vi "BIN_PAQ_content2chunkDefs.vi"(8 "error in (no error)":errorcluster, 11 "Content":string) -> (0 "error out":errorcluster, 3 "Data segments":cluster{"Offset":u32, "Size":u32}[](array[cluster]))   [LabVIEW 2020, in "DBAL-BIN.lvclass"]
doc: "Get PAQ BIN file content and deliver into data chunk segment definitions"
uses:
  DBAL-BIN.lvclass
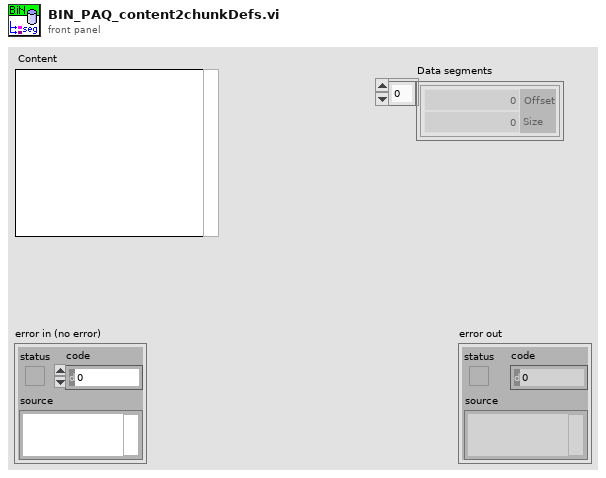
[diagram p1: front panel]
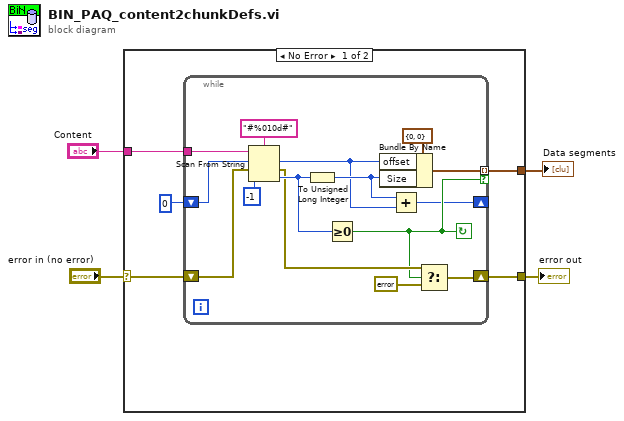
[diagram p0: block diagram]
diagram:
  n1 = case shown="No Error" "error in (no error)" {
    selector: "error in (no error)" -> [w7 w25]
    tunnel: [w6 w25] -> w3
    tunnel: "Content" -> [w9 _]
    tunnel: [w5 _] -> w1
    frame No Error {
      n2 = while {
        tunnel: w9 -> [w18]
        shift-right: [w12] -> _
        shift-left: u32 0 ("offset past scan") -> [w17]
        tunnel: [w22] -> w5 mode=indexing if=w13
        shift-right: [w15] -> w6
        shift-left: w7 -> [w21]
        stop <- w13 continue-if-true
        n3 = Scan From String(format string="#%010d#", input string=w18, initial scan location=w17, error in=w21, default 1=-1 ("default value 1")) -> (offset past scan=w10:u32, error out=w16:errorcluster, output 1=w19:i32)  [unwired: 1 out]
        n4 = To Unsigned Long Integer(number=w19) -> (unsigned 32bit integer=w11:u32)
        n5 = Greater Or Equal To 0?(x=w19) -> (x >= 0?=w13:bool)
        n6 = Bundle By Name(cluster=cluster{"offset":u32, "Size":u32} {"offset"=0, "Size"=0} ("Cluster"), "offset"=w10, "Size"=w11) -> (w22:cluster{"offset":u32, "Size":u32})
        n7 = Add(x=w11, y=w10) -> (x+y=w12:u32)
        n8 = Select(t=w16, s=w13, f=errorcluster {"status"=FALSE, "code"=0, "source"=""}) -> (s? t:f=w15:errorcluster)
      }
    }
    frame Error {
    }
  }
  "error out" <- w3
  "Data segments" <- w1
